vi "Image Display Set ROI Diameter.vi"(8 "Error In":errorcluster, 10 "ROI Diameter":i32=12, 11 "Display Image Control Refnum":T1) -> (0 "Error Out":errorcluster)   [LabVIEW 2021, in "Image.lvlib"]
uses:
  Image.lvlib
  Image Control Refnum.ctl
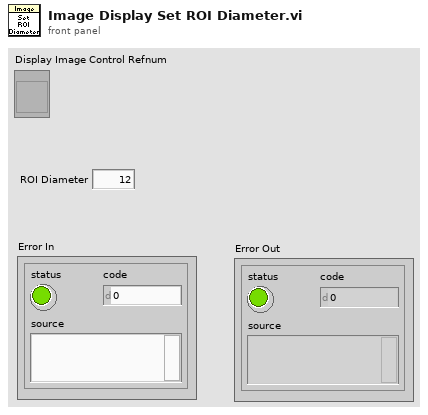
[diagram p1: front panel]
types:
  T1 = typedef "Image.lvlib/Image Control Refnum.ctl" = refnum<vi>
  T2 = cluster{"Global Rectangle":i32[], "Contours":cluster{"Contour Type":u32, "ROI Type":u32, "Points":i32[]}[]}
  T3 = cluster{"Contour Type":u32, "ROI Type":u32, "Points":i32[]}[]
  T4 = cluster{"Contour Type":u32, "ROI Type":u32, "Points":i32[]}
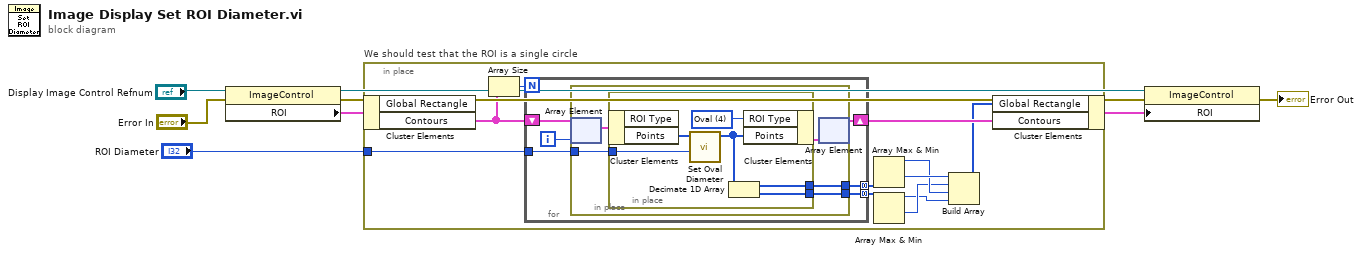
[diagram p0: block diagram]
diagram:
  n1 = property class="ImageControl"(reference="Display Image Control Refnum", error in="Error In") -> (reference out=w4:T1, error out=w3:errorcluster, "ROI"=w6:T2)
  n2 = in-place "We should test that the ROI is a single circle" {
    in-place-border: "ROI Diameter" -> [w19]
    n3 = in-place-cluster #1(w6) -> ("Contours"=w17:T3)  [unwired: 1 out]
    n4 = Array Size(array=w17) -> (size(s)=w16:i32)
    n5 = for {
      N: w16 -> [_]
      tunnel: w19 -> [w25]
      shift-right: [w23] -> w18
      shift-left: w17 -> [w24]
      tunnel: [w21] -> w15 mode=concatenating
      tunnel: [w20] -> w14 mode=concatenating
      i -> [w22]
      n6 = in-place {
        in-place-border: w25 -> [w30]
        in-place-border: [w27] -> w21
        in-place-border: [w26] -> w20
        n7 = in-place-array #2(w24, w22) -> (w29:T4)
        n8 = in-place {
          in-place-border: w30 -> [w34]
          in-place-border: [w32] -> w27
          in-place-border: [w31] -> w26
          w35 = u32 4 items=["No Selection", "Point", "Line", "Rectangle", "Oval", "Polygon", "Freehand Region", "Annulus", "Unused2", "Unused3", "Broken Line", "Freehand Line", "Rotated Rectangle"] ("Type")
          n9 = in-place-cluster #3(w29) -> ("Points"=w36:i32[])  [unwired: 1 out]
          n10 = call "Set Oval Diameter.vi"("ROI Diameter"=w34, "Oval Points in"=w36) -> ("Circle Points out"=w33:i32[])  [unwired: 9 in]
          n11 = Decimate 1D Array(w33) -> (w32:i32[], w31:i32[])
          n12 = in-place-cluster #3("ROI Type"=w35, "Points"=w33) -> (w28:T4)
        }
        n13 = in-place-array #2(w28) -> (w23:T3)  [unwired: 1 out]
      }
    }
    n14 = Array Max & Min(array=w15) -> (max value=w11:i32, min value=w12:i32)  [unwired: 2 out]
    n15 = Array Max & Min(array=w14) -> (max value=w9:i32, min value=w10:i32)  [unwired: 2 out]
    n16 = Build Array(w12, w10, w11, w9) -> (w13:i32[])
    n17 = in-place-cluster #1("Global Rectangle"=w13, "Contours"=w18) -> (w5:T2)
  }
  n18 = property class="ImageControl"(reference=w4, error in=w3, "ROI"=w5) -> (error out=→"Error Out":errorcluster)  [unwired: 1 out]
